vi "RTMain.UpdateVSData.vi"(11 "Refnum in":refnum<k33>) -> (0 "error out":errorcluster)   [LabVIEW 2013, in "OPC UA Client Engine.lvlib"]
uses:
  OPC UA Client Engine.lvlib
  Types/ReadData.Settings
  <vilib>/NI Veristand/Custom Device API/Data Reference.ctl
  <vilib>/NI Veristand/Custom Device API/Global Data Refs.vi
  <vilib>/NI Veristand/Custom Device API/Custom Device API.lvlib
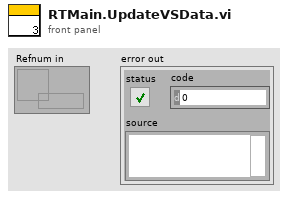
[diagram p1: front panel]
types:
  T1 = typedef "OPC UA Client Engine.lvlib/ReadData.Settings" = cluster{"DataRef":T2, "Value":dbl}
  T2 = typedef "Custom Device API.lvlib/Data Reference.ctl" = i32
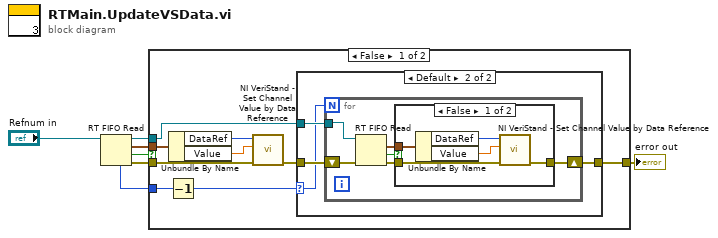
[diagram p0: block diagram]
diagram:
  n1 = RT FIFO Read(0:"Refnum in") -> (7:w1:u32, 8:w6:refnum<k33>, 9:w3:T1, 10:w2:bool, 11:w4:errorcluster)  [unwired: 3 in]
  n2 = case shown="False" w2 {
    tunnel: w1 -> [w12 _]
    tunnel: w3 -> [w16 _]
    tunnel: w4 -> [w15 w34]
    tunnel: [w8 w34] -> w5
    tunnel: w6 -> [w9 _]
    frame False {
      n3 = Decrement(x=w12) -> (x-1=w11:u32)
      n4 = Unbundle By Name(w16) -> ("DataRef"=w14:T2, "Value"=w13:dbl)
      n5 = call <vilib>:"NI VeriStand - Set Channel Value by Data Reference.vi"("error in (no error)"=w15, "Value"=w13, "Data Reference in"=w14) -> ("error out"=w10:errorcluster)  [unwired: 8 in]
      n6 = case shown="Default" w11 {
        selector: w11 -> [_ w18]
        tunnel: w10 -> [w17 w21]
        tunnel: w9 -> [_ w20]
        tunnel: [w17 w19] -> w8
        frame 0 {
        }
        frame Default {
          n7 = for {
            N: w18 -> [_]
            shift-right: [w24] -> w19
            shift-left: w21 -> [w27]
            tunnel: w20 -> [w23]
            n8 = RT FIFO Read(0:w23, 3:w27) -> (9:w25:T1, 10:w22:bool, 11:w26:errorcluster)  [unwired: 2 in, 2 out]
            n9 = case shown="False" w22 {
              tunnel: w26 -> [w30 w33]
              tunnel: w25 -> [w29 _]
              tunnel: [w28 w33] -> w24
              frame False {
                n10 = Unbundle By Name(w29) -> ("DataRef"=w31:T2, "Value"=w32:dbl)
                n11 = call <vilib>:"NI VeriStand - Set Channel Value by Data Reference.vi"("error in (no error)"=w30, "Value"=w32, "Data Reference in"=w31) -> ("error out"=w28:errorcluster)  [unwired: 8 in]
              }
              frame True {
              }
            }
          }
        }
      }
    }
    frame True {
    }
  }
  "error out" <- w5
